vi "DrawCircle.vi"(6 "color(black)":u32(colorbox)=13816530, 9 "pen":T1={"Width"=50, "Style"=enum."Solid"}, 10 "new position":cluster{"x":i16, "y":i16}, 11 "picture":picture) -> (3 "new picture":picture)   [LabVIEW 2023]
doc: "Draws a cross to x and y axis."
panel:
  in  "radius":i16=5
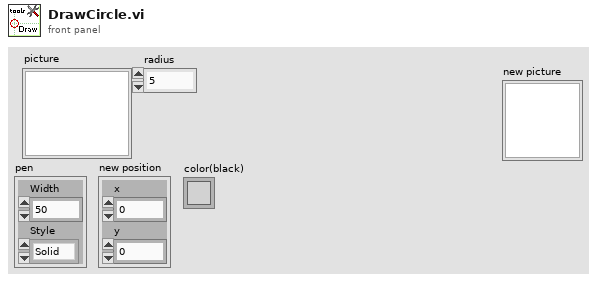
[diagram p1: front panel]
types:
  T1 = cluster{"Width":u16, "Style":enum32{"Solid", "Dash", "Dot", "DashDot", "DashDotDot"}}
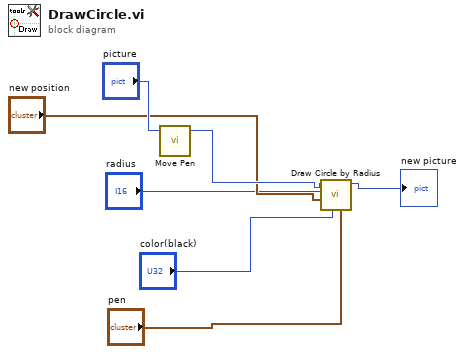
[diagram p0: block diagram]
diagram:
  n1 = call <vilib>:"Move Pen.vi"("picture"="picture") -> ("new picture"=w6:picture)  [unwired: 4 in]
  n2 = call <vilib>:"Draw Circle by Radius.vi"("pen"="pen", "color(black)"="color(black)", "pixel center"="new position", "radius"="radius", "picture"=w6) -> ("new picture"=→"new picture":picture)  [unwired: 6 in]
